vi "CIC_5decimate_4cycles.vi"(7 "reset":bool, 8 "valid in":bool, 11 "Data in":fxp<+/-,16,14>) -> (0 "valid out":bool, 3 "Data out":fxp<+/-,16,14>, 4 "ready for input":bool)   [LabVIEW 2013]
uses:
  <vilib>/rvi/IPIntegrationNode/IPINode_Utilities/niFpgaIPINodeSimCore.vi
  <vilib>/rvi/FXPMathLib/FxpInterpret/XNode/nifxpmath_Interpret.xnode
  <vilib>/rvi/XilinxIP/XIPIN_XNode/niFpgaXIPIN.xnode
  Filters/CIC_5decimate_4cycles/CIC_5decimate_4cycles_65329D8778C1463593165B66C10BC298.dll
  <vilib>/rvi/IPIntegrationNode/IPINode_Xnode/niFpgaIPINode.xnode
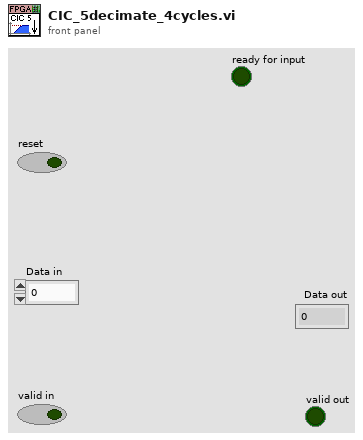
[diagram p1: front panel]
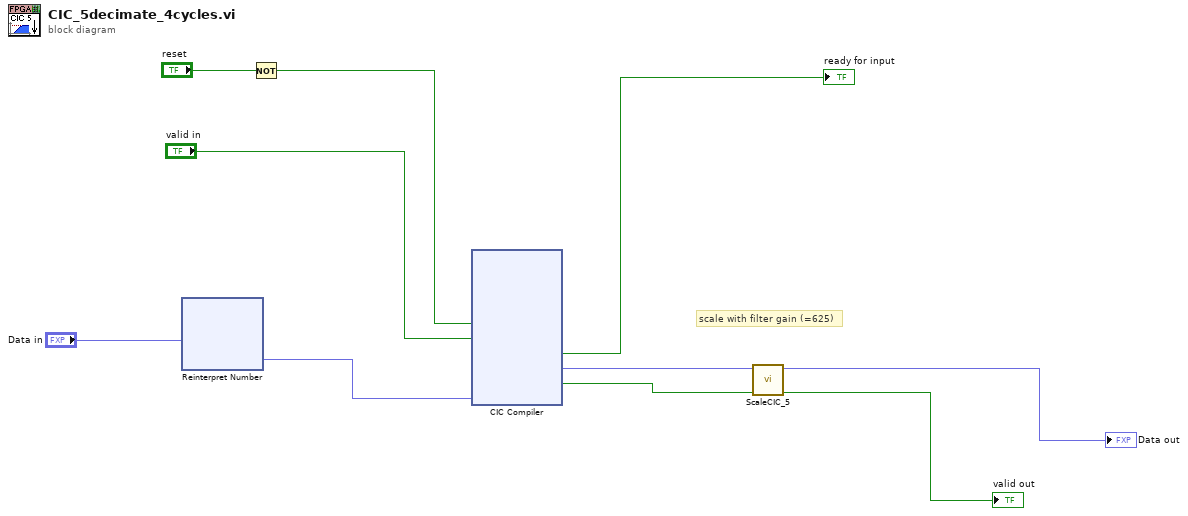
[diagram p0: block diagram]
diagram:
  # "scale with filter gain (=625)"
  n1 = xnode "Reinterpret Number"("x"="Data in") -> ("y"=w5:fxp<+,16,16>)
  n2 = Not(x="reset") -> (.not. x?=w9:bool)
  n3 = xnode ("CIC Compiler")("aresetn"=w9, "s_axis_data_tvalid"="valid in", "s_axis_data_tdata"=w5) -> ("s_axis_data_tready"=→"ready for input":bool, "m_axis_data_tdata"=w4:fxp<+/-,32,32>, "m_axis_data_tvalid"=w3:bool)  [unwired: 1 in]
  n4 = call "ScaleCIC_5.vi"("input valid"=w3, "x"=w4) -> ("valid out"=→"valid out":bool, "Data out"=→"Data out":fxp<+/-,16,14>)  [unwired: 8 in]
